vi "Analog Input Waveform Data.vi"(8 "error in (no error)":errorcluster, 10 "Analog Data":waveform(dbl)[](array[waveform]), 11 "Analog Input Waveform Data in":refnum<class "Analog Input Waveform Data.lvclass">) -> (0 "error out":errorcluster, 3 "Analog Input Waveform Data out":refnum<class "Analog Input Waveform Data.lvclass">)   [LabVIEW 2024, in "DAQmx Actor Interface.lvlib" / "Analog Input Waveform Data.lvclass"]
uses:
  Analog Input Waveform Data.lvclass
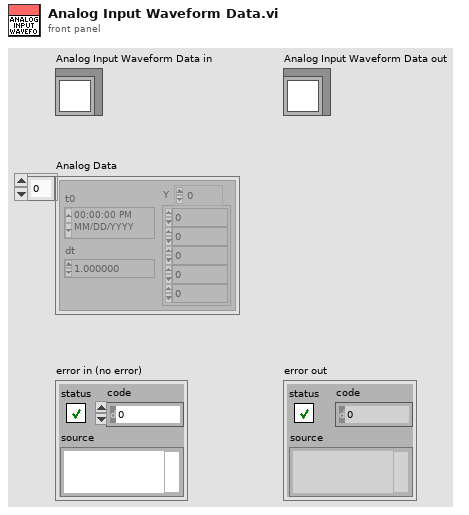
[diagram p1: front panel]
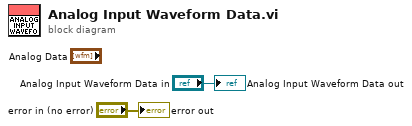
[diagram p0: block diagram]
diagram:
  "error out" <- "error in (no error)"
  "Analog Input Waveform Data out" <- "Analog Input Waveform Data in"
